vi "Get Value By Name.vi"(8 "error in (no error)":errorcluster, 10 "Name":string, 11 "LUT in":refnum<class "LUT.lvclass">) -> (0 "error out":errorcluster, 1 "Value":variant, 2 "found?":bool, 3 "LUT out":refnum<class "LUT.lvclass">)   [LabVIEW 2017, in "LUT.lvlib" / "LUT.lvclass"]
doc: "Returns the corresponding value based on the attribute name."
uses:
  LUT.lvclass
  LUT.lvclass/LUT.ctl
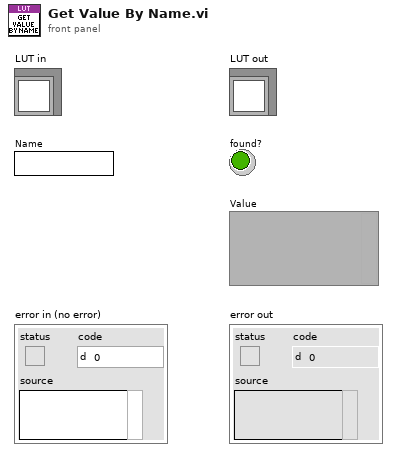
[diagram p1: front panel]
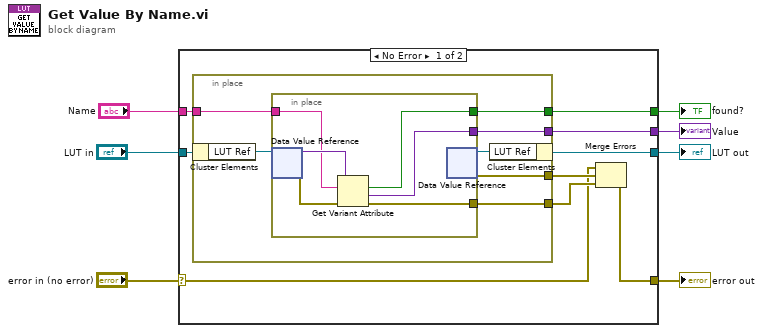
[diagram p0: block diagram]
diagram:
  n1 = case shown="No Error" "error in (no error)" {
    selector: "error in (no error)" -> [w9 w31]
    tunnel: [w8 w31] -> w6
    tunnel: [w15 w30] -> w4
    tunnel: "LUT in" -> [w16 w30]
    tunnel: "Name" -> [w14 _]
    tunnel: [w13 _] -> w2
    tunnel: [w12 _] -> w1
    frame No Error {
      n2 = in-place {
        in-place-border: w14 -> [w21]
        in-place-border: [w20] -> w13
        in-place-border: [w19] -> w12
        in-place-border: [w18] -> w10
        in-place-border: [w17] -> w11
        n3 = in-place-cluster #1(w16) -> ("LUT Ref"=w23:refnum<data-value>)
        n4 = in-place {
          in-place-border: w21 -> [w28]
          in-place-border: [w27] -> w20
          in-place-border: [w26] -> w19
          in-place-border: [w24] -> w18
          n5 = in-place-dvr #2(w23) -> (w29:variant, w25:errorcluster)
          n6 = Get Variant Attribute(Variant=w29, name=w28, error in=w25) -> (found=w26:bool, value=w27:variant, error out=w24:errorcluster)  [unwired: 1 in, 1 out]
          n7 = in-place-dvr #2() -> (w22:refnum<data-value>, w17:errorcluster)  [unwired: 1 in]
        }
        n8 = in-place-cluster #1("LUT Ref"=w22) -> (w15:refnum<class "LUT.lvclass">)
      }
      n9 = Merge Errors(w9, w11, w10) -> (w8:errorcluster)
    }
    frame Error {
    }
  }
  "error out" <- w6
  "LUT out" <- w4
  "Value" <- w2
  "found?" <- w1
